vi "Read Lidar Data (old).vi"(8 "error in (no error)":errorcluster) -> (0 "error out":errorcluster, 3 "Lidar Data":T1={"Directions (rads)"=array[392 elements], "Magnitudes"=[406, 411, 411, 424, 424, 424, 389, 421, 421, 432, 432, 433, 435, 437, 441, 446, 446, 460, 457, 457, 459, 460, 464, 471, 474, 475, 477, 477, 478, 479, 487, 494, 498, 504, 506, 507, 510, 517, 523, 526, 534, 534, 539, 540, 546, 552, 555, 561, 571, 7, 580, 583, 591, 598, 603, 604, 607, 614, 623, 632, 633, 636, 656, 658, 669, 671, 676, 688, 688, 697, 712, 732, 736, 744, 756, 761, 778, 784, 800, 804, 818, 833, 853, 867, 885, 902, 928, 957, 971, 988, 1014, 1036, 1075, 1098, 1114, 1140, 1170, 1187, 1214, 1235, 1258, 1287, 1319, 1338, 1372, 1406, 1456, 1505, 1536, 1605, 1670, 1730, 1872, 16, 0, 0, 0, 0, 0, 0, 2482, 2482, 2482, 2482, 2482, 2478, 2477, 2475, 2475, 2475, 2473, 2470, 2469, 2469, 2432, 2463, 2462, 2460, 2462, 2462, 2459, 2455, 2455, 2455, 2454, 2455, 2455, 2459, 2455, 2459, 2456, 2459, 2459, 2462, 2463, 2463, 2463, 2463, 2465, 2466, 2466, 2468, 2468, 2469, 2474, 2477, 2477, 2482, 2482, 2482, 2483, 2486, 2487, 2490, 2491, 2496, 2497, 38, 2500, 2515, 2516, 2525, 2537, 2537, 2541, 2541, 2543, 2547, 2549, 2549, 2552, 2556, 2557, 2561, 2567, 2576, 2580, 2580, 2599, 2594, 2605, 2613, 2613, 2621, 2624, 2633, 2637, 2649, 2650, 2659, 2667, 2675, 2685, 2690, 2698, 2698, 2716, 2718, 2720, 2737, 2742, 2753, 2762, 2764, 2771, 2778, 2798, 2800, 2803, 2820, 2823, 2842, 2850, 2859, 2867, 2883, 2900, 2907, 2917, 2940, 2949, 42, 2969, 2982, 2996, 3001, 3018, 3030, 3039, 3059, 3069, 3086, 3103, 3113, 3137, 3142, 3163, 3172, 3196, 3217, 3226, 3236, 3246, 3282, 3297, 3311, 3333, 3353, 3373, 3379, 3403, 3425, 3453, 3482, 3482, 3482, 3481, 3464, 3448, 3428, 3411, 3390, 3363, 3349, 3326, 3312, 3292, 3283, 3262, 3244, 3225, 3211, 3207, 3189, 3159, 3159, 3152, 3113, 3091, 3078, 3074, 3067, 3048, 3033, 3016, 51, 2998, 2984, 2970, 2947, 2941, 2934, 2927, 2914, 2909, 2902, 2878, 2864, 2855, 2853, 2846, 2828, 2821, 2810, 2809, 2798, 2798, 2777, 2767, 2764, 2756, 2746, 2742, 2739, 2733, 2716, 2706, 2706, 2705, 2697, 2688, 2684, 2683, 2670, 2659, 2656, 2650, 2647, 2645, 2634, 2632, 2626, 2624, 2614, 2610, 2605, 2602, 2599, 2599, 2590, 2580, 2576, 2575, 2574, 2572, 2571, 2574, 2569, 2566, 41, 2558, 2556, 2556, 2553, 2543, 2543, 2538, 2538, 2538, 2535, 2535, 2535, 2535, 2536, 2540, 2540, 2540, 2546, 2549, 2552, 2600, 2567]})   [LabVIEW 2016]
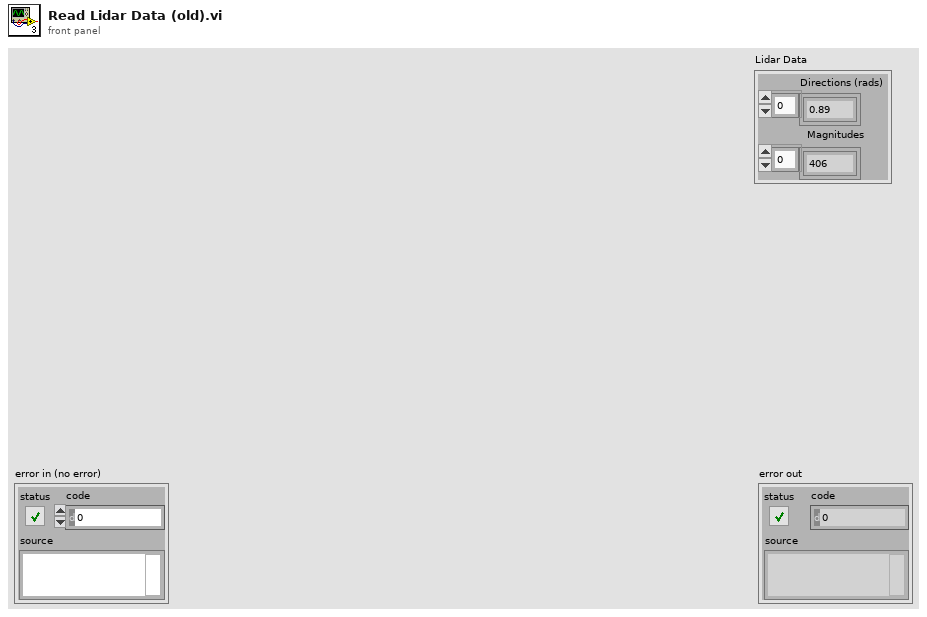
[diagram p1: front panel]
types:
  T1 = cluster{"Directions (rads)":dbl[], "Magnitudes":u16[]}
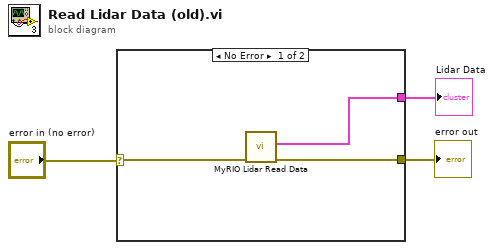
[diagram p0: block diagram]
diagram:
  n1 = case shown="No Error" "error in (no error)" {
    selector: "error in (no error)" -> [w5 w7]
    tunnel: [w6 w7] -> w3
    tunnel: [w4 _] -> w1
    frame No Error {
      n2 = call "MyRIO Lidar Read Data.vi"("error in (no error)"=w5) -> ("error out"=w6:errorcluster, "Lidar Data"=w4:T1)  [unwired: 9 in]
    }
    frame Error {
    }
  }
  "error out" <- w3
  "Lidar Data" <- w1
